vi "Kalman Calculation.vi"(7 "Use Observation":bool=TRUE, 8 "iteração":dbl=1.0, 9 "Pk-1|k-1":T1, 10 "x_k-1|k-1":T1=[[0.0, 0.0, 0.0], [0.0, 0.0, 0.0], [0.0, 0.0, 0.0]], 11 "z_k":T1) -> (1 "SumDiagP":dbl, 2 "Pk|k":T1, 3 "x_k|k":T1)   [LabVIEW 2016]
uses:
  <vilib>/Analysis/Matrix/Datatypes/RealMatrix.ctl
  <vilib>/Analysis/baseanly.llb/Real Inverse Matrix.vi
  <vilib>/Analysis/Matrix/Numeric/Multiply/Multiply - RM,RM.vi
  <vilib>/Analysis/Matrix/Numeric/Add/Add - RM,RM.vi
  <vilib>/Analysis/Matrix/NI_Matrix.lvlib
  <vilib>/Analysis/NI_AALBase.lvlib
panel:
  out "K_k":T1
  out "Inverse Matrix":T1
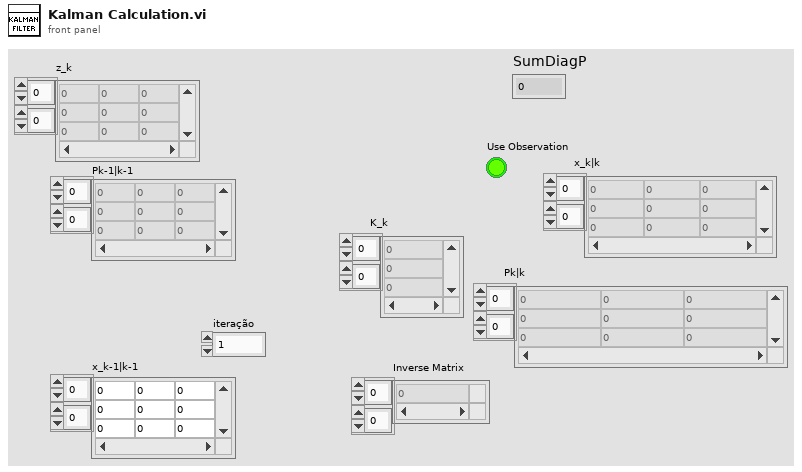
[diagram p1: front panel]
types:
  T1 = typedef "NI_Matrix.lvlib/RealMatrix.ctl" = dbl[][]
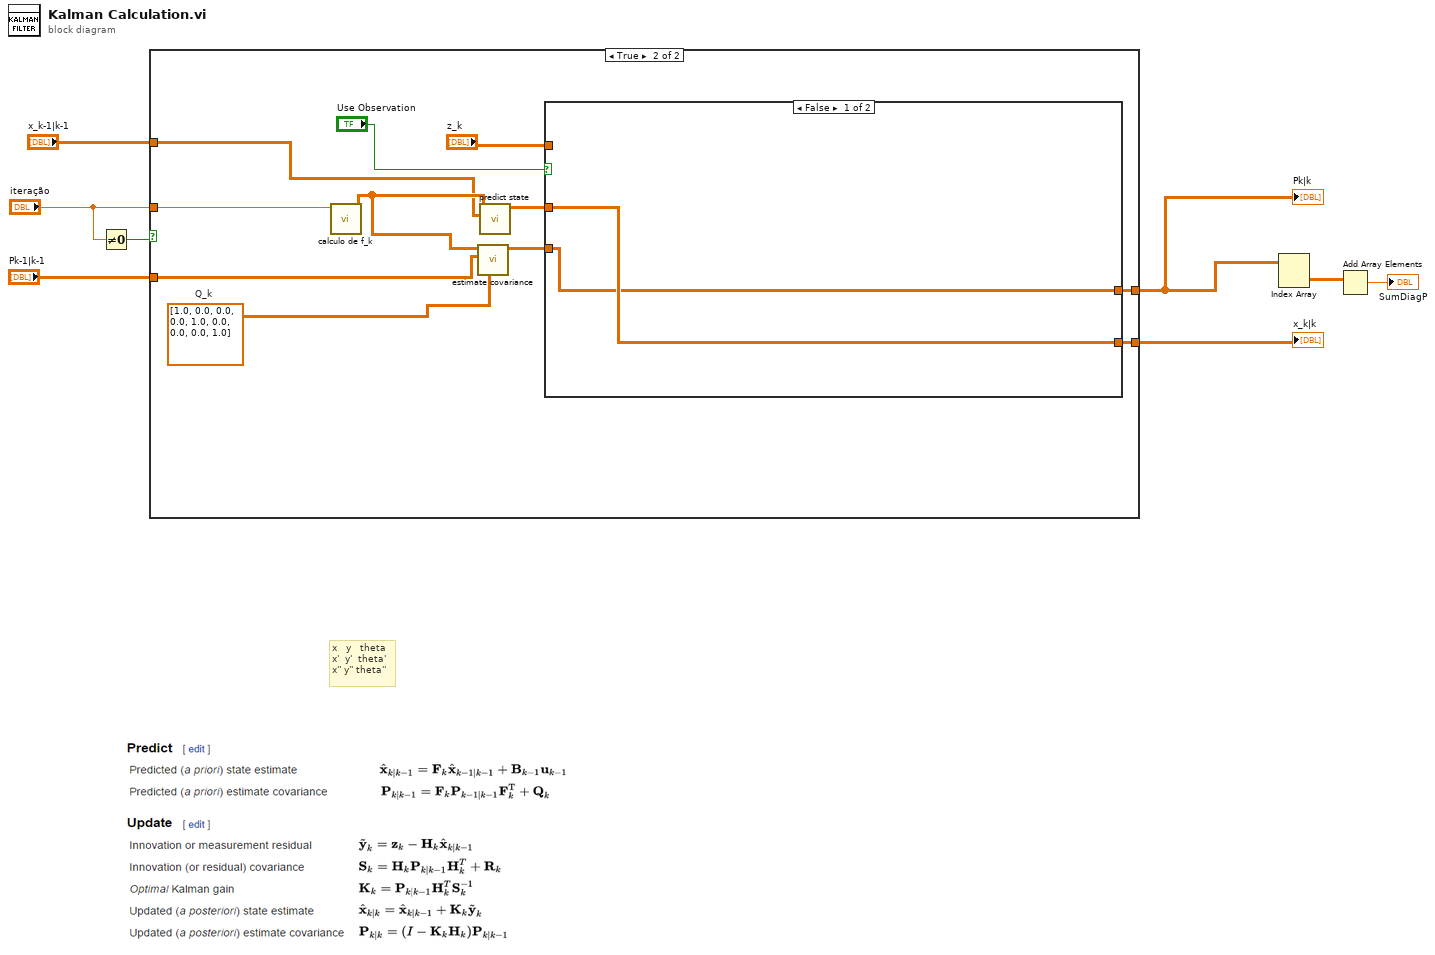
[diagram p0: block diagram]
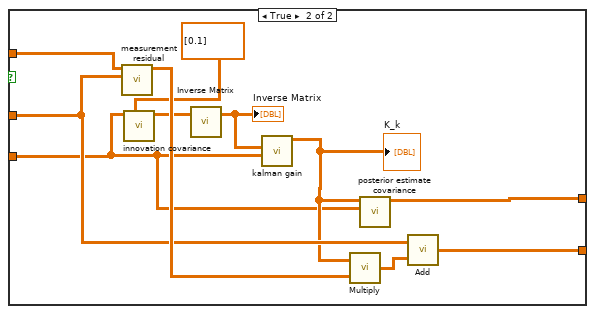
[diagram p3: hidden frame]
diagram:
  # "x   y   theta\nx'  y'  theta'\nx'' y'' theta''"
  n1 = Not Equal To 0?(x="iteração") -> (x != 0?=w2:bool)
  n2 = case shown="True" w2 {
    tunnel: "iteração" -> [_ w21]
    tunnel: [w10 w14] -> w8
    tunnel: "Pk-1|k-1" -> [w9 w13]
    tunnel: "x_k-1|k-1" -> [w10 w12]
    tunnel: [w9 w11] -> w3
    frame False {
    }
    frame True {
      w18 = T1 [[1.0, 0.0, 0.0], [0.0, 1.0, 0.0], [0.0, 0.0, 1.0]]  # Q_k
      n3 = call "calculo de f_k.vi"("iteração"=w21) -> ("F_k"=w20:T1)  [unwired: 10 in]
      n4 = call "estimate covariance.vi"("Q_k"=w18, "Pk-1|k-1"=w13, "F_k"=w20) -> ("Pk|k-1"=w16:T1)  [unwired: 8 in]
      n5 = call "predict state.vi"("x_k-1|k-1"=w12, "F_k"=w20) -> ("x_k|k-1"=w17:T1)  [unwired: 9 in]
      n6 = case shown="False" "Use Observation" {
        tunnel: [w23 w33] -> w14
        tunnel: w17 -> [w23 w31]
        tunnel: [w22 w28] -> w11
        tunnel: w16 -> [w22 w26]
        tunnel: "z_k" -> [_ w24]
        frame False {
        }
        frame True {
          n7 = call "measurement residual.vi"("x_k|k-1"=w31, "z_k"=w24) -> ("y~_k"=w32:T1)  [unwired: 9 in]
          n8 = call "innovation covariance.vi"("R"=T1 [[0.1]], "Pk|k-1"=w26) -> ("S_k"=w30:T1)  [unwired: 8 in, 1 out]
          n9 = call-poly <vilib>:"Inverse Matrix.vi"("Input Matrix"=w30) -> ("Inverse Matrix"=w29:T1)  [unwired: 1 in, 1 out]
          "Inverse Matrix" <- w29
          n10 = call "kalman gain.vi"("Pk|k-1"=w26, "S^-1"=w29) -> ("K_k"=w27:T1)  [unwired: 9 in]
          "K_k" <- w27
          n11 = call-poly <vilib>:"Multiply.vi"("Real Matrix B"=w32, "Real Matrix A"=w27) -> ("A * B"=w34:T1)
          n12 = call "posterior estimate covariance.vi"("Pk|k-1"=w26, "K_k"=w27) -> ("Pk|k"=w28:T1)  [unwired: 9 in]
          n13 = call-poly <vilib>:"Add.vi"("Real Matrix B"=w34, "Real Matrix A"=w31) -> ("A + B"=w33:T1)
        }
      }
    }
  }
  "x_k|k" <- w8
  "Pk|k" <- w3
  n14 = Index Array(array=w3) -> (element=w7:T1)  [unwired: 2 in]
  n15 = Add Array Elements(numeric array=w7) -> (sum=→"SumDiagP":dbl)
